vi "Validate_Proper Indentation.vi"(0 "Functions in":T1[](array[typedef]), 11 "error in (no error)":errorcluster) -> (4 "Functions":T1[](array[typedef]), 6 "Validation message":T2[](array[typedef]), 15 "error out":errorcluster)   [LabVIEW 2019, in "LSL.lvlib" / "scripts manager.lvclass"]
uses:
  scripts manager.lvclass
  common/line and indent/Line Details.ctl
  common/function utils/Validate_message.ctl
  common/function utils/Validate_MessageStatus.ctl
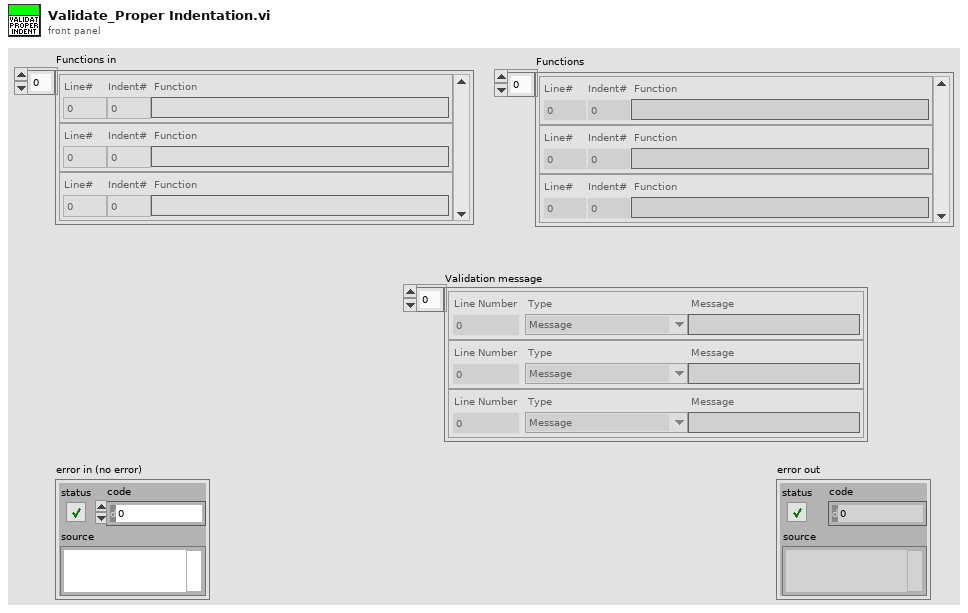
[diagram p1: front panel]
types:
  T1 = typedef "Line Details.ctl" = cluster{"Line#":i64, "Indent#":i64, "Function":string}
  T2 = typedef "Validate_message.ctl" = cluster{"Line Number":i64, "Type":T3, "Message":string}
  T3 = typedef "Validate_MessageStatus.ctl" = enum16{"Message", "Warning", "Error"}
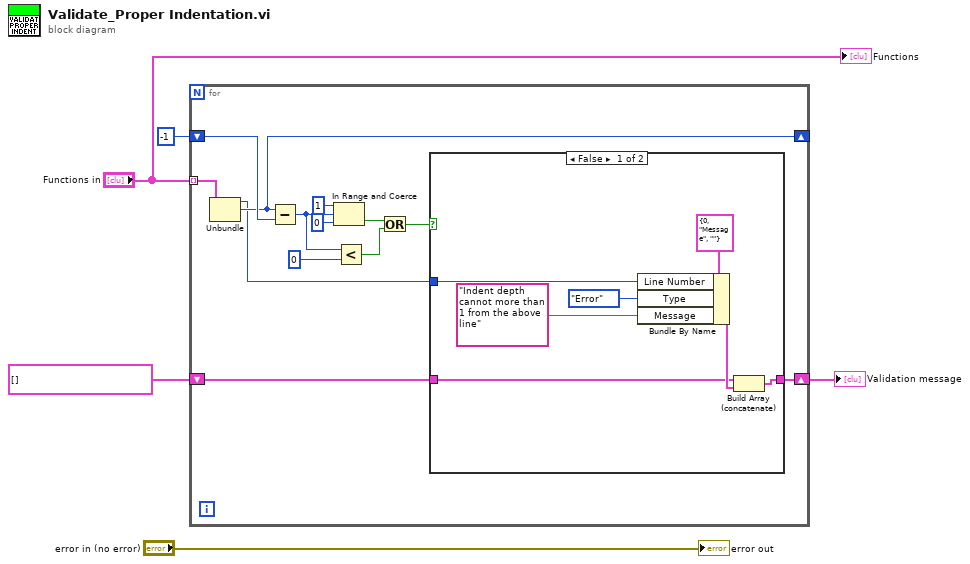
[diagram p0: block diagram]
diagram:
  n1 = for {
    tunnel: "Functions in" -> [w12] mode=indexing
    shift-right: [w10] -> _
    shift-left: i64 -1 ("Indent") -> [w18]
    shift-right: [w7] -> w1
    shift-left: T2[] [] -> [w6]
    n2 = Unbundle(w12) -> ("Line#"=w9:i64, "Indent#"=w10:i64)  [unwired: 1 out]
    n3 = Subtract(x=w10, y=w18) -> (x-y=w8:i64)
    n4 = In Range and Coerce(upper limit=i64 1, x=w8, lower limit=i64 0) -> (In Range?=w14:bool)  [unwired: 1 out]
    n5 = Less?(x=w8, y=i64 0) -> (x < y?=w13:bool)
    n6 = Or(x=w14, y=w13) -> (x .or. y?=w11:bool)
    n7 = case shown="False" w11 {
      tunnel: w9 -> [w24 _]
      tunnel: [w21 w26] -> w7
      tunnel: w6 -> [w20 w26]
      frame False {
        n8 = Bundle By Name(cluster=T2 {"Line Number"=0, "Type"=enum."Message", "Message"=""} ("Message"), "Line Number"=w24, "Type"=Validate_MessageStatus."Error", "Message"="Indent depth cannot more than 1 from the above line") -> (w22:T2)
        n9 = Build Array (concatenate)(w20, w22) -> (w21:T2[])
      }
      frame True {
      }
    }
  }
  "Validation message" <- w1
  "error out" <- "error in (no error)"
  "Functions" <- "Functions in"
